vi "Replace Test.vi"() -> ()   [LabVIEW 2017]
uses:
  <vilib>/gpm_packages/@cs/linked-list/Source/Linked List/Linked List/Linked List.lvclass
  C:/Program Files/National Instruments/LabVIEW 2017/vi.lib/gpm_packages/@cs/linked-list/Source/Linked List/ILinkedList/ILinked List.lvclass
  29df65f9-43f5-4274-83e8-a4d57e3390a8.vi
  b1a18c1f-f0fd-4297-a1ac-b8d99e6db1c0.vi
  <vilib>/gpm_packages/@cs/linked-list/Source/Linked List/ILinkedList/ILinked List.lvclass
  <vilib>/gpm_packages/@cs/linked-list/Source/Linked List/Linked List Ref/Linked List Ref.lvclass
panel:
  out "Child IDs":string[](array[string])
  in  "Tree 2":string(tree)
  in  "Tree":string(tree)
  out "Replaced?":bool
  out "Attribute":string
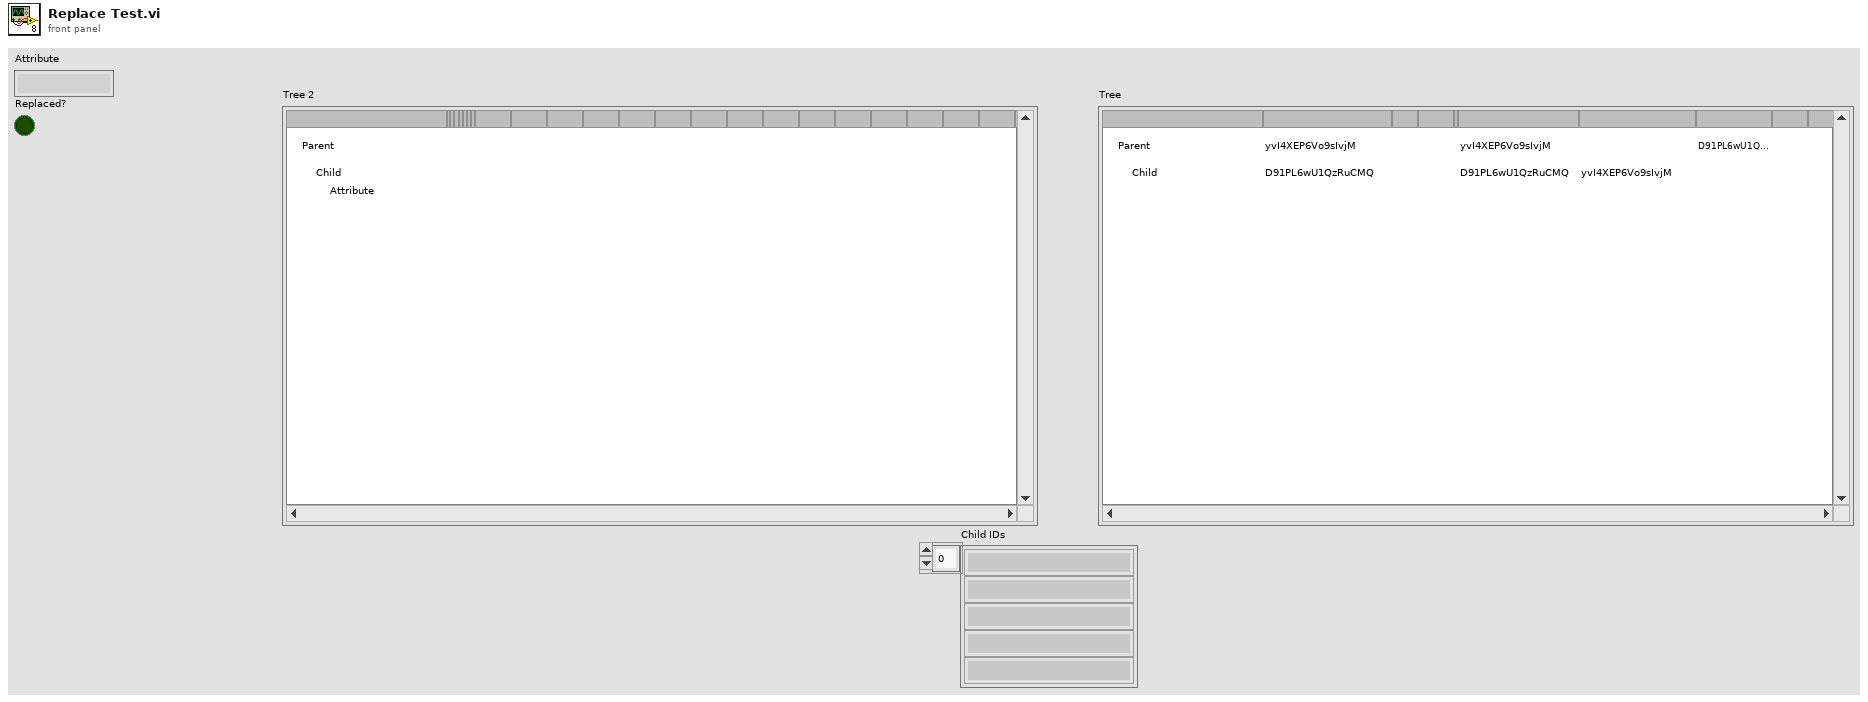
[diagram p1: front panel]
types:
  T1 = cluster{"Left Cell String":string, "Child Text":string[], "Child Tag":string, "Item Indent":i32, "Child Only?":bool, "Glyph Index":i32}[]
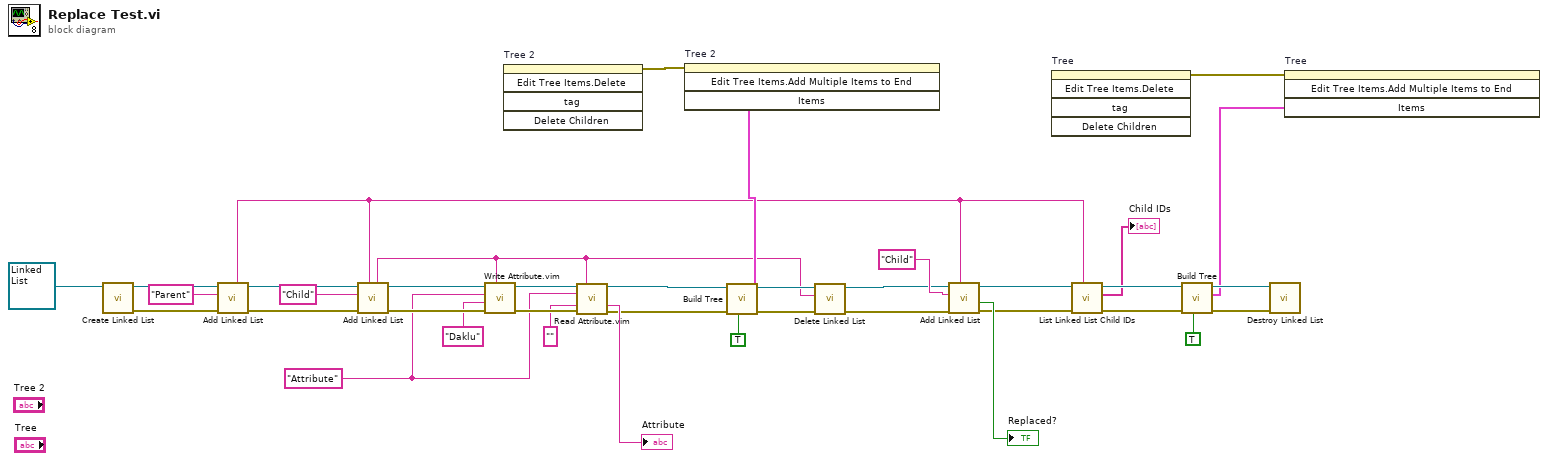
[diagram p0: block diagram]
diagram:
  w25 = "Attribute" ("Attribute Name")
  n1 = call <vilib>:"Create Linked List.vi"("Linked List"=refnum<class "Linked List.lvclass"> refnum ("Linked Lists.lvlib:Linked List.lvclass")) -> ("error out"=w36:errorcluster, "Linked List Ref"=w37:refnum<data-value>)  [unwired: 9 in]
  n2 = call <vilib>:"Add Linked List.vi"("error in (no error)"=w36, "Name"="Parent", "Linked List Ref"=w37) -> ("error out"=w33:errorcluster, "Linked List Ref out"=w34:refnum<data-value>, "Linked List ID out"=w2:string)  [unwired: 5 in, 1 out]
  n3 = call <vilib>:"Add Linked List.vi"("Parent ID"=w2, "error in (no error)"=w33, "Name"="Child", "Linked List Ref"=w34) -> ("error out"=w31:errorcluster, "Linked List Ref out"=w32:refnum<data-value>, "Linked List ID out"=w7:string)  [unwired: 4 in, 1 out]
  n4 = call "Write Attribute.vim"("Linked List ID"=w7, "error in (no error)"=w31, "Attribute"="Daklu" ("Attribute Name"), "Attribute Name"=w25, "Linked List Ref"=w32) -> ("error out"=w28:errorcluster, "Linked List Ref out"=w29:refnum<data-value>)  [unwired: 3 in, 2 out]
  n5 = invoke on="Tree 2" class="Tree (strict)" method="Edit Tree Items.Delete"() -> (error out=w14:errorcluster)  [unwired: 5 in, 4 out]
  n6 = call "Read Attribute.vim"("Linked List Ref"=w29, "Linked List ID"=w7, "Attribute Name"=w25, "Type"="", "error in (no error)"=w28) -> ("Linked List Ref out"=w17:refnum<data-value>, "Attribute"=→"Attribute":string, "error out"=w16:errorcluster)  [unwired: 5 in, 3 out]
  n7 = call <vilib>:"Build Tree.vi"("Show IDs"=TRUE, "error in (no error)"=w16, "Linked List Ref"=w17) -> ("error out"=w9:errorcluster, "Tree Data"=w15:T1, "Linked List Ref out"=w11:refnum<data-value>)  [unwired: 6 in]
  n8 = invoke on="Tree 2" class="Tree (strict)" method="Edit Tree Items.Add Multiple Items to End"(error in=w14, "Items"=w15) -> ()  [unwired: 2 in, 4 out]
  n9 = call <vilib>:"Delete Linked List.vi"("error in (no error)"=w9, "Linked List ID"=w7, "Linked List Ref"=w11) -> ("error out"=w8:errorcluster, "Linked List Ref out"=w10:refnum<data-value>)  [unwired: 7 in]
  n10 = call <vilib>:"Add Linked List.vi"("Parent ID"=w2, "error in (no error)"=w8, "Name"="Child", "Linked List Ref"=w10) -> ("error out"=w4:errorcluster, "Replaced?"=→"Replaced?":bool, "Linked List Ref out"=w6:refnum<data-value>)  [unwired: 4 in, 1 out]
  n11 = invoke on="Tree" class="Tree (strict)" method="Edit Tree Items.Delete"() -> (error out=w19:errorcluster)  [unwired: 5 in, 4 out]
  n12 = call <vilib>:"List Linked List Child IDs.vi"("Linked List ID"=w2, "error in (no error)"=w4, "Linked List Ref"=w6) -> ("error out"=w3:errorcluster, "Child IDs"=→"Child IDs":string[], "Linked List Ref out"=w5:refnum<data-value>)  [unwired: 6 in]
  n13 = call <vilib>:"Build Tree.vi"("Show IDs"=TRUE, "error in (no error)"=w3, "Linked List Ref"=w5) -> ("error out"=w23:errorcluster, "Tree Data"=w21:T1, "Linked List Ref out"=w22:refnum<data-value>)  [unwired: 6 in]
  n14 = call <vilib>:"Destroy Linked List.vi"("error in (no error)"=w23, "Linked List Ref"=w22) -> ()  [unwired: 9 in, 1 out]
  n15 = invoke on="Tree" class="Tree (strict)" method="Edit Tree Items.Add Multiple Items to End"(error in=w19, "Items"=w21) -> ()  [unwired: 2 in, 4 out]
